vi "Get PDOMapping.vi"(11 "ODentry in":refnum<class "ODentry.lvclass">) -> (2 "PDOMapping":bool, 3 "ODentry out":refnum<class "ODentry.lvclass">)   [LabVIEW 2024, in "EDS.lvlib" / "ODentry.lvclass"]
uses:
  ODentry.lvclass
  ODentry.lvclass/ODentry.ctl
  PDO Mapping Type.ctl
  EDS.lvlib
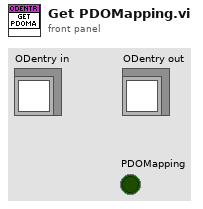
[diagram p1: front panel]
types:
  T1 = typedef "EDS.lvlib/PDO Mapping Type.ctl" = enum16{"NO", "OPTIONAL", "RPDO", "TPDO", "@DEFAULT"}
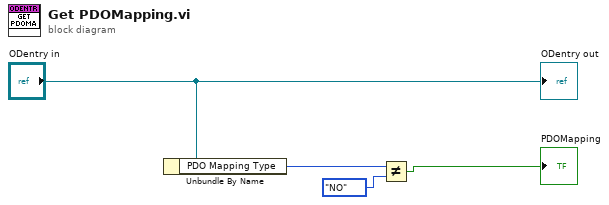
[diagram p0: block diagram]
diagram:
  n1 = Unbundle By Name("ODentry in") -> ("PDO Mapping Type"=w3:T1)
  n2 = Not Equal?(x=w3, y=PDO_Mapping_Type."NO" ("PDO Mapping Type")) -> (x != y?=→"PDOMapping":bool)
  "ODentry out" <- "ODentry in"
